vi "Filter Event Data.vi"(8 "error in (no error)":errorcluster, 10 "EventFilter Reference":T1, 11 "EventDataMessage in":refnum<class "EventDataMessage.lvclass">) -> (0 "error out":errorcluster, 2 "Discard?":bool, 3 "EventDataMessage out":refnum<class "EventDataMessage.lvclass">)   [LabVIEW 2017, in "ActorEvents.lvlib" / "EventDataMessage.lvclass"]
uses:
  EventDataMessage.lvclass
  IEventFilter/EventFilter Reference.ctl
  IEventFilter/IEventFilter.lvclass
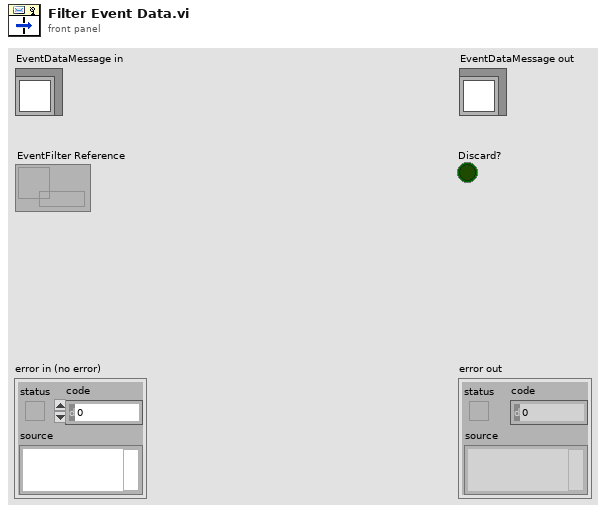
[diagram p1: front panel]
types:
  T1 = typedef "ActorEvents.lvlib/IEventFilter.lvclass/EventFilter Reference.ctl" = refnum<data-value>
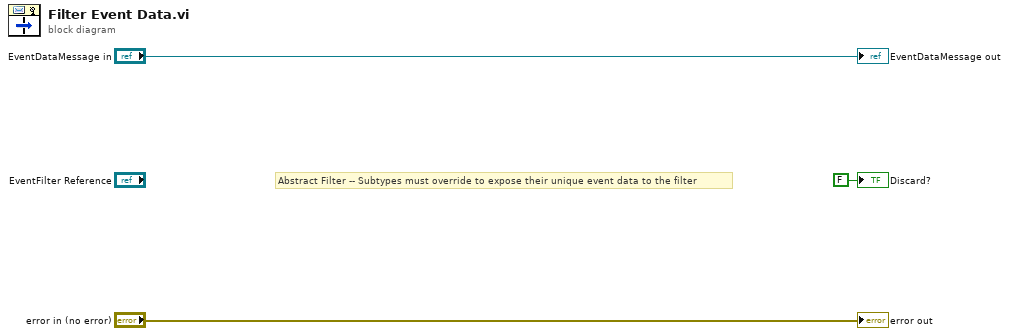
[diagram p0: block diagram]
diagram:
  # "Abstract Filter -- Subtypes must override to expose their unique event data to the filter"
  "error out" <- "error in (no error)"
  "EventDataMessage out" <- "EventDataMessage in"
  "Discard?" <- FALSE ("Discard?")
